vi "Globals.vi"() -> ()   [LabVIEW 2014]
panel:
  out "SCMP":enum16{"COMP", "SCD"}(ring)
  in  "comp collision arrea":dbl[](array[numeric])=[27.0, 27.0, 27.0, 21.0]
  in  "scd max range":dbl[](array[numeric])=[154.0, 1.0, 1.0]
  in  "comp max range":dbl[](array[numeric])=[27.0, 27.0, 21.0]
  in  "scd parking pos":dbl[](array[numeric])=[100.0, 0.0, 0.0]
  out "first power on":bool
  in  "comp parking pos":dbl[](array[numeric])=[20.0, 20.0, 20.0]
  in  "FITS BITPIX":enum16{"16", "32"}(ring)
  # "//float PI_12   kolizia cam1 s cam2\n//float PI_13;  kolizia cam1 s cam3,4\n//float PI_21;  kolizia cam2 s cam1\n//float PI_31;  kolizia cam3,4 s cam1"
  # "mh jul2020\nPI_13 by malo byt okolo 25\n-davam ale na 27 aby neboli hlasky collision area\n-zaroven max range pre PI3 26->21"
  # "jr 20200320:\n  allowed PI position intervals: ANDOR T [0.1 - +27.0] mm\n  without a collision ANDOR R [0.1 - +27.0] mm\n                                 GOOODRICH [0.1 - +26.0] mm"
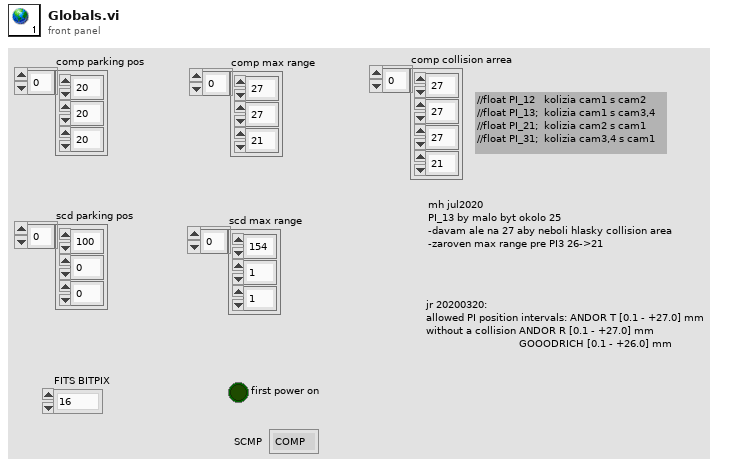
[diagram p1: front panel]
diagram:
